vi "SelectStriptestProber.vi"() -> ()   [LabVIEW 2013]
panel:
  out "Number of Strips:":string
  in  "Cancel Button":bool
  in  "Start":bool
  in  "Eject Button":bool
  in  "Chuck":bool caption="Chuck\nDOWN"
  in  "Overdrive [µm]":i32=30
  in  "Speed [µm/step]":i32=20
  in  "Search Band [µm]":i32=100
  # "Probestation"
  # "Edgesense"
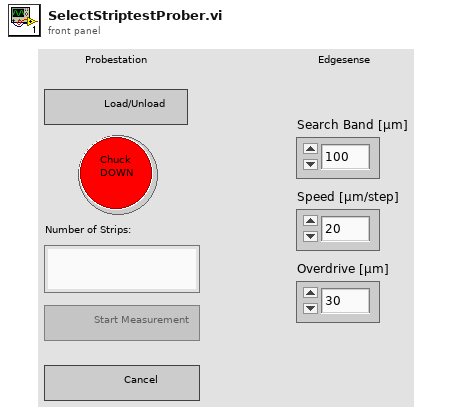
[diagram p1: front panel]
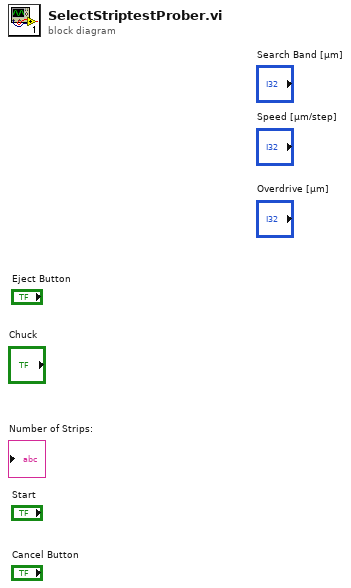
[diagram p0: block diagram]
diagram:
